vi "Quick Start - Simple - Upload File.vi"(11 "File Path":path) -> ()   [LabVIEW 2020]
doc: "CSV File Path: Path to the local CSV file.\nDataset Name: Desired name for the dataset on Nominal.\nTimestamp Column: Name of the timestamp column in your CSV file.\nTimestamp Type: Type of timestamp (e.g., Epoch or ISO8601).\nDescription (optional): Text description for the dataset.\nWait Until Complete (optional): Whether to wait for ingestion completion."
uses:
  Nominal Client/Nominal Client.lvclass/Nominal Client.ctl
  datasources/dataset/dataset.lvclass
  nominal types/channelConfig/channelConfig.lvclass
  7453b450-11aa-4de2-86c8-e10972c9b5f7.vi
  88f255ab-c32d-4dd6-bf15-c9130b619246.vi
  ec386b0f-4bc9-4d19-a6ff-1680e8debb9b.vi
  Nominal Client/private_data.set.vi
  datasources/s3/s3.lvclass
  C:/code/labview-client/lv_src/datasources/source/source.lvclass
  <vilib>/Utility/file.llb/Application Directory.vi
  <vilib>/Utility/error.llb/Error Cluster From Error Code.vi
  Nominal Client/upload_ingest.csv.vi
  datasources/source/create_s3.vi
  ts.iso8601/build.iso8601.vi
  datasources/target/create_new.vi
  Nominal Client/ingest_csv.vi
  Nominal Client/catalog.wait_until_ingest_complete.vi
  Nominal Client/Nominal Client.lvclass
  nominal types/workspace/workspace.lvclass
  submodules/reqwest-labview/lv-src/reqwest/reqwest.lvclass
  timestampMetadata/timestampMetadata.lvclass
  datasources/target/target.lvclass
  datasources/source/source.lvclass
  ts.iso8601/ts.iso8601.lvclass
  C:/code/labview-client/lv_src/datasources/payload/payload.lvclass
  C:/code/labview-client/lv_src/datasources/s3/s3.lvclass
panel:
  in  "Use Express Method":bool
  in  "Labels":string[](array[string])
  in  "Property Name":string[](array[string])
  in  "Property Value":string[](array[string])
  in  "Wait Until Complete":bool
  in  "Description":string
  in  "Timestamp Column Name":string
  in  "Dataset Name":string
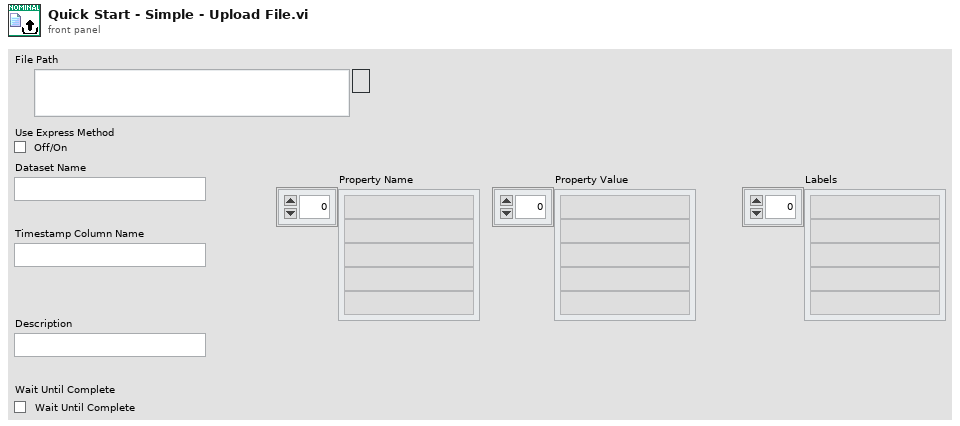
[diagram p1: front panel]
types:
  T1 = cluster{"dataset":refnum<class "dataset.lvclass">, "channelConfig":refnum<class "channelConfig.lvclass">}
  T2 = cluster{"channelPrefix":string, "tagKeysFromColumns":string[], "tagColums":map{string, string}, "additionalFileTags":map{string, string}}
  T3 = cluster{"Property Name":string[], "Property Value":string[]}
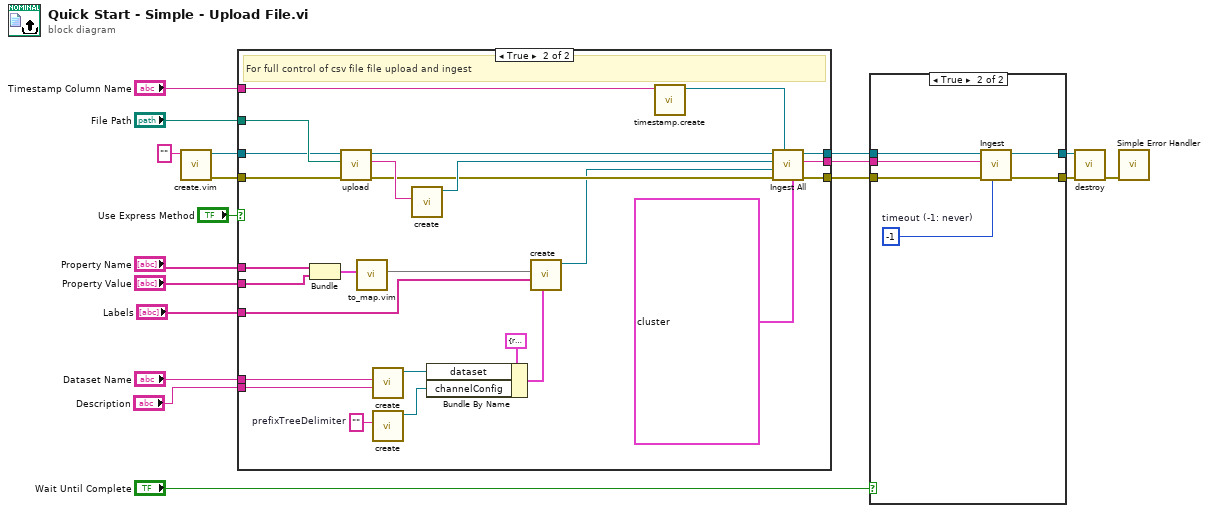
[diagram p0: block diagram]
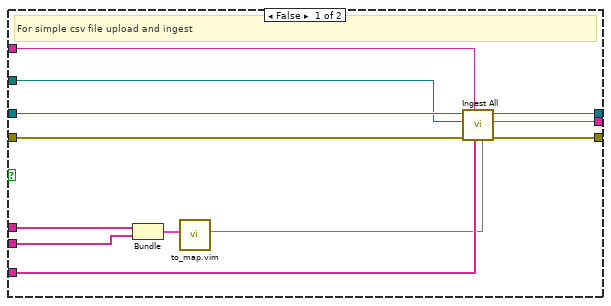
[diagram p2: hidden frame]
diagram:
  n1 = call "create.vim"("API Token (string or path)"="") -> ("error out"=w8:errorcluster, "Nominal Client"=w9:refnum<class "Nominal Client.lvclass">)  [unwired: 9 in]
  n2 = case shown="True" "Use Express Method" {
    tunnel: "Property Name" -> [w21 w56]
    tunnel: "Property Value" -> [w20 w55]
    tunnel: "Timestamp Column Name" -> [w24 w53]
    tunnel: "File Path" -> [w25 w52]
    tunnel: w9 -> [w28 w51]
    tunnel: w8 -> [w27 w50]
    tunnel: [w29 w48] -> w7
    tunnel: [w26 w47] -> w6
    tunnel: [w30 w46] -> w5
    tunnel: "Labels" -> [w23 w38]
    tunnel: "Dataset Name" -> [_ w37]
    tunnel: "Description" -> [_ w36]
    frame False {
      # "For simple csv file upload and ingest"
      n3 = Bundle("Property Name"=w21, "Property Value"=w20) -> (w22:T3)  [unwired: 1 in]
      n4 = call "to_map.vim"("Map"=w22) -> ("Map out"=w19:map{string, string})  [unwired: 10 in]
      n5 = call-poly "Ingest All.vi"("Properties"=w19, "Labels"=w23, "Timestamp SeriesName"=w24, "error in"=w27, "File Path"=w25, "Nominal Client in"=w28) -> ("error out"=w30:errorcluster, "datasetRID"=w26:string, "Nominal Client out"=w29:refnum<class "Nominal Client.lvclass">)  [unwired: 3 in]
    }
    frame True {
      w31 = ""  # prefixTreeDelimiter
      # "For full control of csv file file upload and ingest"
      n6 = Bundle("Property Name"=w56, "Property Value"=w55) -> (w54:T3)  [unwired: 1 in]
      n7 = call "upload.vi"("error in"=w50, "File"=w52, "Nominal Client in"=w51) -> ("error out"=w42:errorcluster, "Path to S3 File"=w44:string, "Nominal Client out"=w49:refnum<class "Nominal Client.lvclass">)  [unwired: 6 in]
      n8 = call "to_map.vim"("Map"=w54) -> ("Map out"=w39:map{string, string})  [unwired: 10 in]
      n9 = call "create.vi"("Description"=w36, "Name"=w37) -> ("dataset"=w34:refnum<class "dataset.lvclass">)  [unwired: 9 in]
      n10 = call "create.vi"("prefixTreeDelimiter"=w31) -> ("channelConfig"=w32:refnum<class "channelConfig.lvclass">)  [unwired: 10 in]
      n11 = call-poly "create.vi"("Path"=w44) -> ("source"=w43:refnum<class "s3.lvclass">)  [unwired: 10 in]
      n12 = Bundle By Name(cluster=T1 {"dataset"=refnum, "channelConfig"=refnum} ("Optional"), "dataset"=w34, "channelConfig"=w32) -> (w33:T1)
      n13 = call-poly "create.vi"("Optional"=w33, "Labels"=w38, "Properties"=w39) -> ("New Target"=w40:refnum<class "target.lvclass">)  [unwired: 8 in]
      n14 = call-poly "timestamp.create.vi"("seriesName"=w53) -> ("Timestamp Metadata"=w45:refnum<class "timestampMetadata.lvclass">)  [unwired: 10 in]
      n15 = call-poly "Ingest All.vi"("optional"=T2 {"channelPrefix"="", "tagKeysFromColumns"=[], "tagColums"={}, "additionalFileTags"={}}, "timestampMetadata"=w45, "error in"=w42, "Target"=w40, "Source"=w43, "Nominal Client in"=w49) -> ("error out"=w46:errorcluster, "datasetRid"=w47:string, "Nominal Client out"=w48:refnum<class "Nominal Client.lvclass">)  [unwired: 2 in, 1 out]
    }
  }
  n16 = case shown="True" "Wait Until Complete" {
    tunnel: w7 -> [w57 w64]
    tunnel: w5 -> [w58 w63]
    tunnel: [w58 w62] -> w17
    tunnel: [w57 w61] -> w16
    tunnel: w6 -> [_ w60]
    frame False {
    }
    frame True {
      w59 = -1  # timeout (-1: never)
      n17 = call-poly "Ingest.vi"("timeout (-1: never)"=w59, "error in"=w63, "datasetRid"=w60, "Nominal Client"=w64) -> ("error out"=w62:errorcluster, "Nominal Client out"=w61:refnum<class "Nominal Client.lvclass">)  [unwired: 6 in]
    }
  }
  n18 = call "destroy.vi"("error in"=w17, "Nominal Client"=w16) -> ("error out"=w14:errorcluster)  [unwired: 9 in]
  n19 = call <vilib>:"Simple Error Handler.vi"("error in (no error)"=w14) -> ()  [unwired: 4 in, 5 out]
